vi "Get Pre Amp Gain.vi"(8 "error in (no error)":errorcluster, 10 "gain":sgl, 11 "index":i32) -> (0 "error out":errorcluster, 2 "gain out":sgl, 3 "function return":u32)   [LabVIEW 2014, in "atmcd32d.lvlib"]
doc: "unsigned int WINAPI GetPreAmpGain(int index, float * gain);"
uses:
  atmcd32d.lvlib
  atmcd32d.dll
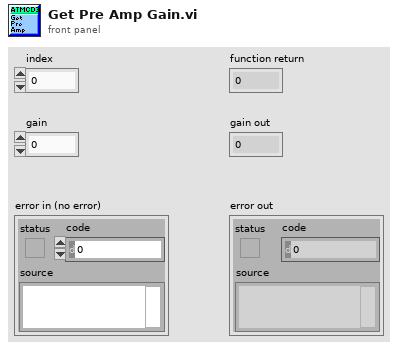
[diagram p1: front panel]
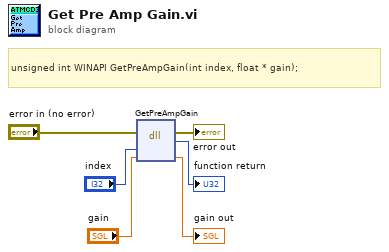
[diagram p0: block diagram]
diagram:
  # "unsigned int WINAPI GetPreAmpGain(int index, float * gain);"
  n1 = dll-call lib="C:/Users/Bakir/Documents/Lambda2-Testing/lib/Andorlib/atmcd32d.*" fn="GetPreAmpGain"(error in="error in (no error)", "index"="index", "gain"="gain") -> (error out=→"error out":errorcluster, →"function return":u32, "gain"=→"gain out":sgl)  [unwired: 3 in, 1 out]
